vi "MES_POST.vi"(7 "DATA":string, 8 "错误输入（无错误）":errorcluster, 11 "URL":string) -> (0 "错误输出":errorcluster, 1 "headers":string caption="头部", 2 "body":string)   [LabVIEW 2015]
uses:
  <vilib>/httpClient/POSTBuffer.vi
  <vilib>/httpClient/LabVIEWHTTPClient.lvlib
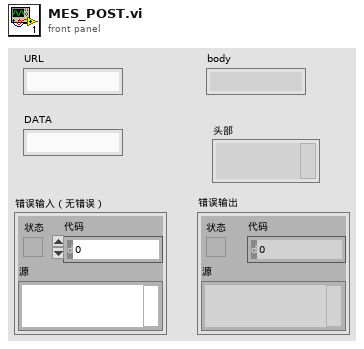
[diagram p1: front panel]
types:
  T1 = typedef "LabVIEWHTTPClient.lvlib/ClientHandle.ctl" = refnum<k1>
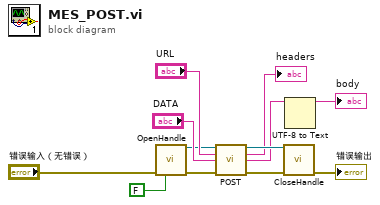
[diagram p0: block diagram]
diagram:
  n1 = call <vilib>:"OpenHandle.vi"("error in (no error)"="错误输入（无错误）", "verify server(true)"=FALSE) -> ("client handle out"=w2:T1, "error out"=w1:errorcluster)  [unwired: 12 in]
  n2 = call-poly <vilib>:"POST.vi"("client handle"=w2, "url"="URL", "buffer"="DATA", "error in (no error)"=w1) -> ("client handle out"=w9:T1, "headers"=→"headers":string, "body"=w4:string, "error out"=w8:errorcluster)  [unwired: 8 in]
  n3 = call <vilib>:"CloseHandle.vi"("client handle"=w9, "error in (no error)"=w8) -> ("error out"=→"错误输出":errorcluster)  [unwired: 13 in]
  n4 = UTF-8 to Text(11:w4) -> (3:→"body":string)  [unwired: 2 in, 1 out]
